vi "test-DiffDrvPoseEst2-Test1.vi"(8 "error in (no error)":errorcluster) -> (0 "error out":errorcluster, 3 "Test Passed":bool)   [LabVIEW 2019]
uses:
  <vilib>/Rock Robotics/WPI/ThirdParty/JAS_Junk/TrajLib/Rotation2d_CreateAngle.vi
  <vilib>/Rock Robotics/WPI/ThirdParty/JAS_Junk/TrajLib/Translation2d_Create.vi
  <vilib>/Rock Robotics/WPI/ThirdParty/JAS_Junk/TrajLib/MatBuilder_Create.vi
  <vilib>/Rock Robotics/SystemInterfaces/NetworkCommunication/NetComm_UsageReport_report.vi
  <vilib>/Rock Robotics/WPI/ThirdParty/JAS_Junk/TrajLib/Globals/Util_LibraryGlobals.vi
  <vilib>/Rock Robotics/WPI/ThirdParty/JAS_Junk/TrajLib/Trajectory_Library.lvlib
panel:
  out "Sub error":bool
  out "End Y pos passed":bool
  out "End X pos passed":bool
  out "AddVisionCount":i32
  out "TotalTImeSecs 2":dbl
  out "BenchProcessing \nTimer Per Pass":dbl
  out "BenchTotalTime":dbl
  out "BenchTotalPasses":dbl
  out "MaxErrPassed":bool
  out "MeanPassed":bool
  out "ErrorSumNormalized":dbl
  out "Error Sum":dbl
  out "Max Error":dbl
  out "VIsionMeasCount":i32
  out "TotalTImeSecs":dbl
  out "Position Graph":cluster{dbl[], dbl[]}[](graph)
  out "PoseEst2NewErr":errorcluster
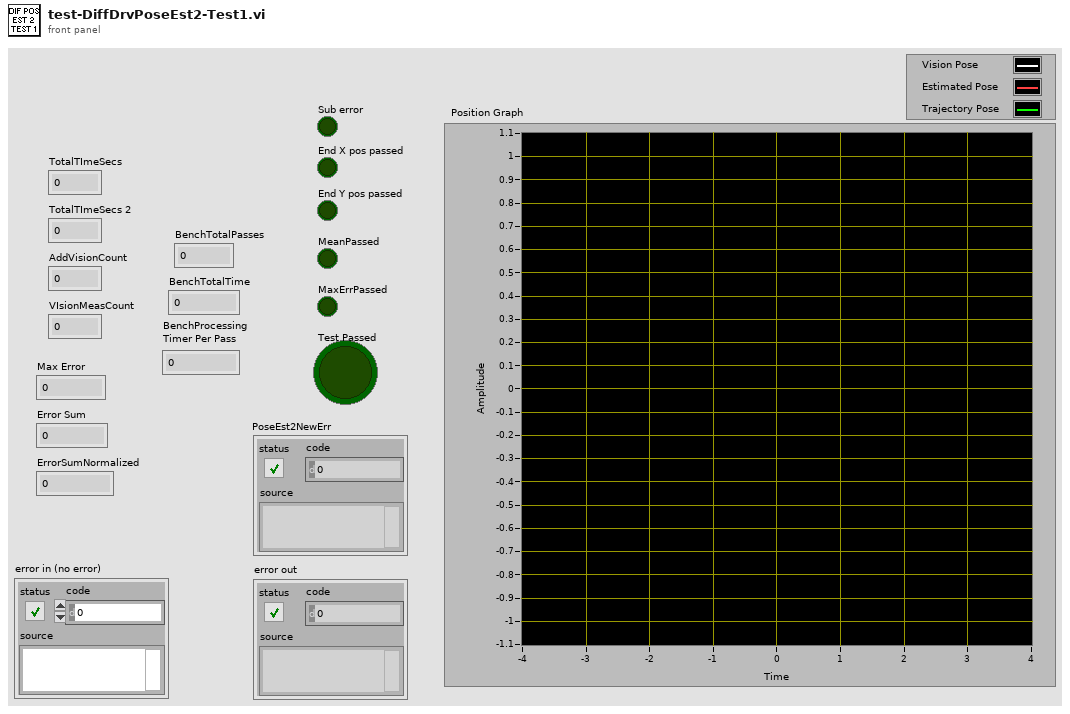
[diagram p1: front panel]
types:
  T1 = typedef "Trajectory_Library.lvlib/POSE2D.ctl" = cluster{"TRANSLATION":T2, "ROTATION":T3}
  T2 = typedef "Trajectory_Library.lvlib/TRANSLATION2D.ctl" = cluster{"X":dbl, "Y":dbl}
  T3 = typedef "Trajectory_Library.lvlib/ROTATION2D.ctl" = cluster{"VALUE":dbl, "COS":dbl, "SIN":dbl}
  T4 = typedef "NI_Matrix.lvlib/RealMatrix.ctl" = dbl[][]
  T5 = typedef "Trajectory_Library.lvlib/TRAJ_CONFIG.ctl" = cluster{"MaxVelocity":dbl, "Max Acceleration":dbl, "StartVelocity":dbl, "End Velocity":dbl, "Reversed":bool, "Constraints":variant[]}
  T6 = typedef "Trajectory_Library.lvlib/DIFF_DRIVE_KINEMATICS.ctl" = cluster{"TrackWidth_Meters":dbl}
  T7 = typedef "Trajectory_Library.lvlib/DIFF_DRIVE_POSE_EST2.ctl" = cluster{"M_Vision_K":T4, "m_nominal_dT":dbl, "m_PrevTime_Sec":dbl, "Pose_Buffer":T8, "Diff_Drive_Kinematics":T6, "Diff_Drive_Odom_2":T9, "M_Q":T4}
  T8 = typedef "Trajectory_Library.lvlib/TIME_INTERPOLATABLE_VARIANT.ctl" = cluster{"TimeStamps":dbl[], "DataArray":variant[], "Min_TimeStamp":dbl, "Max_TimeStamp":dbl, "ItemCount":i32, "MaxBufferTime":dbl}
  T9 = typedef "Trajectory_Library.lvlib/DIFF_DRIVE_ODOM2.ctl" = cluster{"M_POSE_Meters":T1, "M_GyroOffset":T3, "M_PrevAngle":T3, "M_PrevLeftDist_M":dbl, "M_PrevRightDist_M":dbl, "M_InitLeftDist_M":dbl, "M_InitRightDist_M":dbl}
  T10 = typedef "Trajectory_Library.lvlib/TRAJECTORY.ctl" = cluster{"TotalTImeSecs":dbl, "States":T11[]}
  T11 = typedef "Trajectory_Library.lvlib/TRAJ_STATE.ctl" = cluster{"TimeSeconds":dbl, "Velocity":dbl, "Acceleration":dbl, "POSE":T1, "Curvature":dbl}
  T12 = cluster{"MaxErrPassed":bool, "MeanPassed":bool, "Error Sum":dbl, "ErrorSumNormalized":dbl, "Max Error":dbl, "AddVisionCount":i32, "VIsionApplyCount":i32, "BenchTotalPasses":dbl, "BenchTotalTime":dbl, "BenchProcessing \nTimer Per Pass":dbl, "TotalTImeSecs":dbl, "End X pos passed":bool, "End Y pos passed":bool, "Sub error":bool}
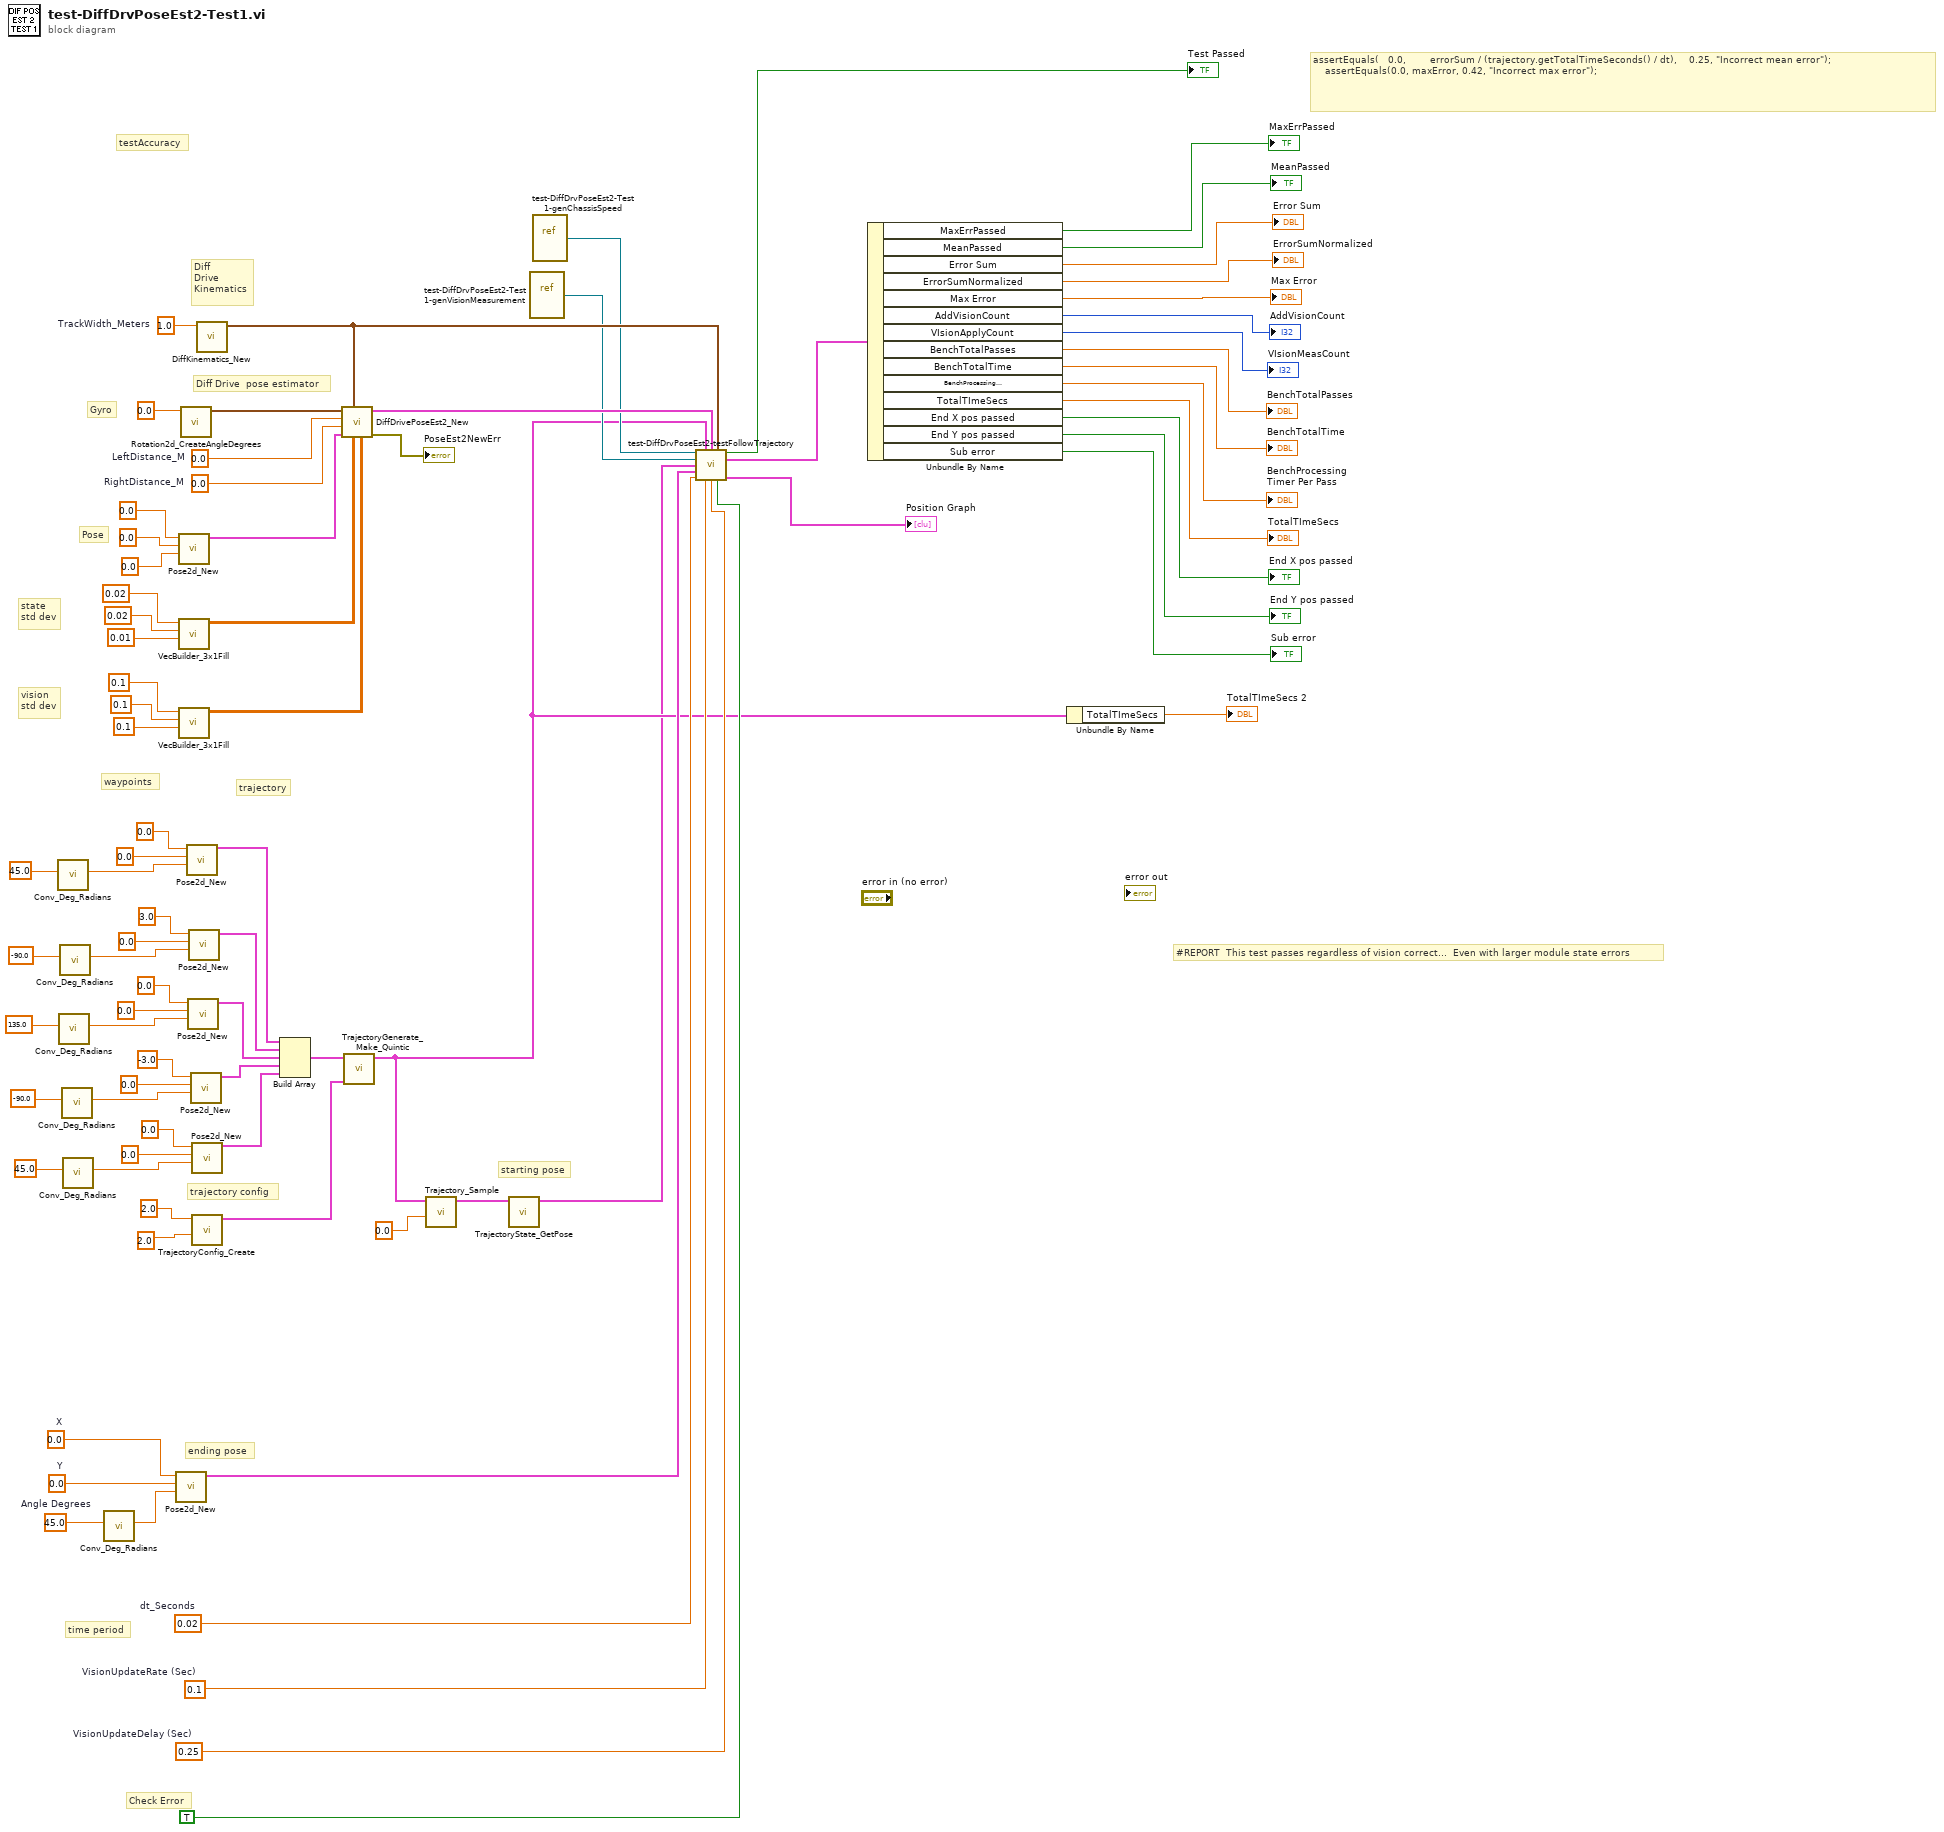
[diagram p0: block diagram]
diagram:
  w27 = 0.25  # VisionUpdateDelay (Sec)
  w28 = 0.1  # VisionUpdateRate (Sec)
  w33 = 0.0  # X
  w32 = 0.0  # Y
  w30 = 45.0  # Angle Degrees
  w41 = 1.0  # TrackWidth_Meters
  w44 = 0.0  # RightDistance_M
  w45 = 0.0  # LeftDistance_M
  w34 = 0.02  # dt_Seconds
  # "testAccuracy"
  # "starting pose"
  # "Check Error"
  # "ending pose"
  # "state \nstd dev"
  # "Diff\nDrive\nKinematics"
  # "#REPORT  This test passes regardless of vision correct...  Even with larger module state errors"
  # "assertEquals(   0.0,        errorSum / (trajectory.getTotalTimeSeconds() / dt),    0.25, \"Incorrect mean error\");\n    assertEquals(0.0, maxError, 0.42, \"Incorrect max error\");"
  # "time period"
  # "vision \nstd dev"
  # "Pose"
  # "Gyro"
  # "Diff Drive  pose estimator"
  # "trajectory config"
  # "trajectory"
  # "waypoints"
  n1 = call <vilib>:"Conv_Deg_Radians.vi"("Degress"=45.0 ("Heading")) -> ("Radians"=w59:dbl)  [unwired: 10 in]
  n2 = call <vilib>:"Conv_Deg_Radians.vi"("Degress"=135.0 ("Heading")) -> ("Radians"=w67:dbl)  [unwired: 10 in]
  n3 = call <vilib>:"Conv_Deg_Radians.vi"("Degress"=-90.0 ("Heading")) -> ("Radians"=w63:dbl)  [unwired: 10 in]
  n4 = call <vilib>:"Conv_Deg_Radians.vi"("Degress"=-90.0 ("Heading")) -> ("Radians"=w71:dbl)  [unwired: 10 in]
  n5 = call <vilib>:"Conv_Deg_Radians.vi"("Degress"=45.0 ("Heading")) -> ("Radians"=w75:dbl)  [unwired: 10 in]
  n6 = call <vilib>:"Conv_Deg_Radians.vi"("Degress"=w30) -> ("Radians"=w31:dbl)  [unwired: 10 in]
  n7 = call <vilib>:"Pose2d_New.vi"("Heading"=w31, "Y"=w32, "X"=w33) -> ("out POSe"=w29:T1)  [unwired: 8 in]
  n8 = call <vilib>:"Pose2d_New.vi"("Heading"=0.0, "Y"=0.0, "X"=0.0) -> ("out POSe"=w43:T1)  [unwired: 8 in]
  n9 = call <vilib>:"VecBuilder_3x1Fill.vi"("R2"=0.01 ("element"), "R1"=0.02 ("element"), "R0"=0.02 ("element")) -> ("output matrix"=w37:T4)  [unwired: 8 in]
  n10 = call <vilib>:"VecBuilder_3x1Fill.vi"("R2"=0.1 ("element"), "R1"=0.1 ("element"), "R0"=0.1 ("element")) -> ("output matrix"=w36:T4)  [unwired: 8 in]
  n11 = call <vilib>:"Rotation2d_CreateAngleDegrees.vi"("Angle_Degrees"=0.0) -> ("ROTATION"=w42:T3)  [unwired: 10 in]
  n12 = call <vilib>:"Pose2d_New.vi"("Heading"=w59, "Y"=0.0, "X"=0.0) -> ("out POSe"=w58:T1)  [unwired: 8 in]
  n13 = call <vilib>:"Pose2d_New.vi"("Heading"=w67, "Y"=0.0, "X"=0.0) -> ("out POSe"=w55:T1)  [unwired: 8 in]
  n14 = call <vilib>:"Pose2d_New.vi"("Heading"=w63, "Y"=0.0, "X"=3.0) -> ("out POSe"=w56:T1)  [unwired: 8 in]
  n15 = call <vilib>:"Pose2d_New.vi"("Heading"=w71, "Y"=0.0, "X"=-3.0) -> ("out POSe"=w54:T1)  [unwired: 8 in]
  n16 = call <vilib>:"Pose2d_New.vi"("Heading"=w75, "Y"=0.0, "X"=0.0) -> ("out POSe"=w80:T1)  [unwired: 8 in]
  n17 = call <vilib>:"TrajectoryConfig_Create.vi"("MaxAcceleration"=2.0, "MaxVelocity"=2.0) -> ("TRAJECTORY_CONFIG"=w77:T5)  [unwired: 9 in]
  n18 = call <vilib>:"DiffKinematics_New.vi"("TrackWidth_Meters"=w41) -> ("DIFF_DRIVE_KINEMATICS"=w24:T6)  [unwired: 10 in]
  n19 = Build Array(w58, w56, w55, w54, w80) -> (w78:T1[])
  n20 = call <vilib>:"DiffDrivePoseEst2_New.vi"("VisionMeasurementStdDevs"=w36, "StateStdDevs"=w37, "DIFF_DRIVE_KINEMATICS"=w24, "InitialPose"=w43, "RightDistance_M"=w44, "LeftDistance_M"=w45, "gyroAngle"=w42) -> ("Error"=→"PoseEst2NewErr":errorcluster, "DiffDrivePoseEstimate"=w35:T7)  [unwired: 3 in]
  n21 = call <vilib>:"TrajectoryGenerate_Make_Quintic.vi"("traj_config"=w77, "waypointPOSE"=w78) -> ("TRAJECTORY"=w5:T10)  [unwired: 8 in, 1 out]
  n22 = call <vilib>:"Trajectory_Sample.vi"("Time"=0.0, "InputTRAJECTORY"=w5) -> ("OutputTRAJ_STATE"=w3:T11)  [unwired: 9 in]
  n23 = call <vilib>:"TrajectoryState_GetPose.vi"("TRAJ_STATE"=w3) -> ("TrajStatePose"=w2:T1)  [unwired: 10 in]
  n24 = vi-ref "test-DiffDrvPoseEst2-Test1-genVisionMeasurement.vi"() -> (w22:refnum<vi>)
  n25 = vi-ref "test-DiffDrvPoseEst2-Test1-genChassisSpeed.vi"() -> (w23:refnum<vi>)
  n26 = call "test-DiffDrvPoseEst2-testFollowTrajectory.vi"("chassisSpeedsGenerator"=w23, "TRAJECTORY"=w5, "DiffDrivePoseEstimate"=w35, "DIFF_DRIVE_KINEMATICS"=w24, "genVisionMeasurement"=w22, "StartingPose"=w2, "EndingPose"=w29, "dt_Seconds"=w34, "VisionUpdateRate"=w28, "VisionUpdateDelay"=w27, "CheckError"=TRUE) -> ("Test Passed"=→"Test Passed":bool, "Output Data"=w19:T12, "DataForGraph"=→"Position Graph":cluster{dbl[], dbl[]}[])  [unwired: 2 in]
  n27 = Unbundle By Name(w19) -> ("MaxErrPassed"=→"MaxErrPassed":bool, "MeanPassed"=→"MeanPassed":bool, "Error Sum"=→"Error Sum":dbl, "ErrorSumNormalized"=→"ErrorSumNormalized":dbl, "Max Error"=→"Max Error":dbl, "AddVisionCount"=→"AddVisionCount":i32, "VIsionApplyCount"=→"VIsionMeasCount":i32, "BenchTotalPasses"=→"BenchTotalPasses":dbl, "BenchTotalTime"=→"BenchTotalTime":dbl, "BenchProcessing \nTimer Per Pass"=→"BenchProcessing \nTimer Per Pass":dbl, "TotalTImeSecs"=→"TotalTImeSecs":dbl, "End X pos passed"=→"End X pos passed":bool, "End Y pos passed"=→"End Y pos passed":bool, "Sub error"=→"Sub error":bool)
  n28 = Unbundle By Name(w5) -> ("TotalTImeSecs"=→"TotalTImeSecs 2":dbl)
